vi "SE Initialization VI.vi"(8 "error in (no error)":errorcluster, 10 "Custom XML":string, 11 "Device Item Ref in":T1 format="%.0x") -> (0 "error out":errorcluster, 3 "Device Item Ref out":T1 format="%.0x")   [LabVIEW 2012, in "PXImc System Explorer.lvlib"]
uses:
  PXImc System Explorer.lvlib
  <vilib>/NI Veristand/Custom Device API/Custom Device Item Ref.ctl
  <vilib>/NI Veristand/Custom Device API/Custom Device Channel Type.ctl
  Shared/Channel.ctl
  Shared/Constants.vi
  <vilib>/dlg_ctls.llb/Space Constant.vi
  Shared/PXImc Shared.lvlib
  <vilib>/NI Veristand/Custom Device API/Custom Device API.lvlib
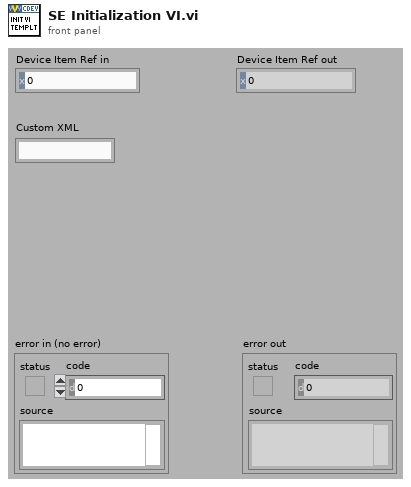
[diagram p1: front panel]
types:
  T1 = typedef "Custom Device API.lvlib/Custom Device Item Ref.ctl" = u64
  T2 = typedef "Custom Device API.lvlib/Custom Device Channel Type.ctl" = enum16{"Input", "Output"}
  T3 = typedef "PXImc Shared.lvlib/Channel.ctl" = cluster{"Name":string, "Units":string, "Default":dbl, "Description":string}
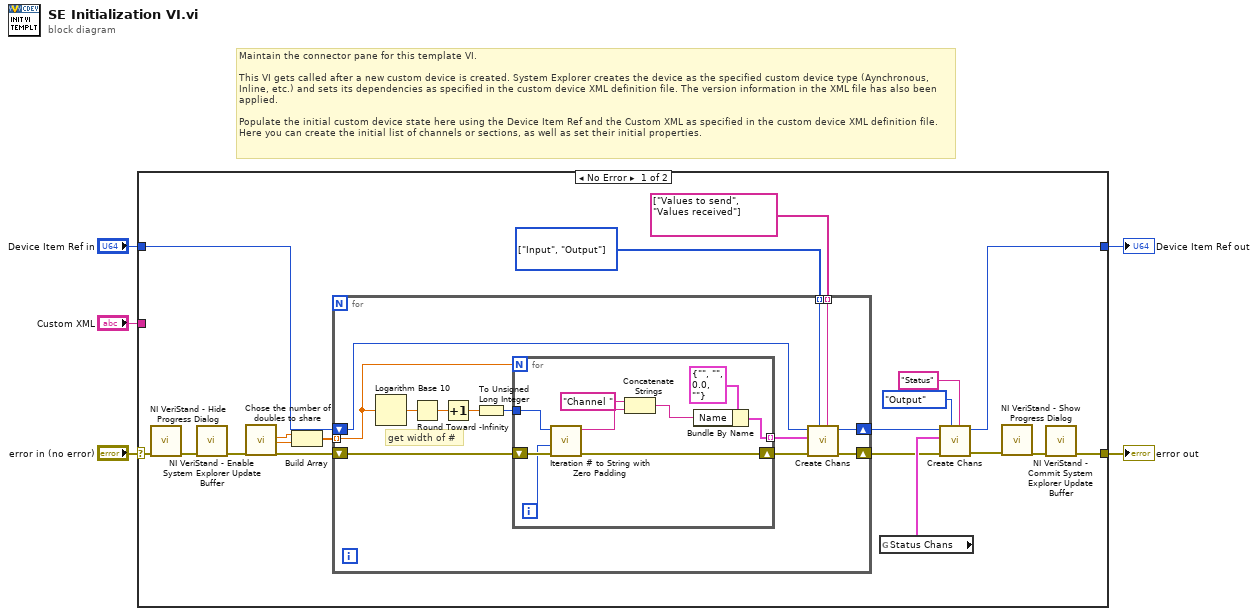
[diagram p0: block diagram]
diagram:
  # "Maintain the connector pane for this template VI.\n\nThis VI gets called after a new custom device is created. System Explorer creates the device as the specified custom device type (Aynchronous, Inline, etc.) and sets its dependencies as specified in the custom device XML definition file. The version information in the XML file has also been applied.\n\nPopulate the initial custom device state here using the Device Item Ref and the Custom XML as specified in the custom device XML definition file. Here you can create the initial list of channels or sections, as well as set their initial properties."
  n1 = case shown="No Error" "error in (no error)" {
    selector: "error in (no error)" -> [w17 w48]
    tunnel: [w12 w48] -> w5
    tunnel: [w24 w47] -> w3
    tunnel: "Device Item Ref in" -> [w10 w47]
    tunnel: "Custom XML" -> [_ _]
    frame No Error {
      w7 = T2[] [enum."Input", enum."Output"] items=["Input", "Output"]
      n2 = call <vilib>:"NI VeriStand - Hide Progress Dialog.vi"("error in (no error)"=w17) -> ("error out"=w16:errorcluster)  [unwired: 10 in]
      n3 = call <vilib>:"NI VeriStand - Enable System Explorer Update Buffer.vi"("error in (no error)"=w16) -> ("error out"=w15:errorcluster)  [unwired: 10 in]
      n4 = call "Chose the number of doubles to share"("error in (no error)"=w15) -> ("Doubles to receive"=w20:dbl, "Doubles to send"=w21:dbl, "error out"=w18:errorcluster)  [unwired: 15 in, 1 out]
      n5 = Build Array(w20, w21) -> (w19:dbl[])
      n6 = for {
        tunnel: w19 -> [w26] mode=indexing
        shift-right: [w36] -> w11
        shift-left: w18 -> [w37]
        shift-right: [w33] -> w9
        shift-left: w10 -> [w34]
        tunnel: string[] ["Values to send", "Values received"] -> [w31] mode=indexing
        tunnel: w7 -> [w30] mode=indexing
        # "get width of #"
        n7 = Logarithm Base 10(1:w26) -> (0:w27:dbl)
        n8 = Round Toward -Infinity(1:w27) -> (0:w28:dbl)
        n9 = Increment(x=w28) -> (x+1=w29:dbl)
        n10 = To Unsigned Long Integer(number=w29) -> (unsigned 32bit integer=w25:u32)
        n11 = for {
          N: w26 -> [_]
          shift-right: [w41] -> w35
          shift-left: w37 -> [w44]
          tunnel: [w45] -> w32 mode=indexing
          tunnel: w25 -> [w43]
          i -> [w42]
          n12 = call "Iteration # to String with Zero Padding.vi"("error in (no error)"=w44, "Current #"=w42, "Width"=w43) -> ("error out"=w41:errorcluster, "String"=w39:string)  [unwired: 7 in]
          n13 = Concatenate Strings("Channel " ("string"), w39) -> (w38:string)
          n14 = Bundle By Name(cluster=T3 {"Name"="", "Units"="", "Default"=0.0, "Description"=""} ("Channel"), "Name"=w38) -> (w45:T3)
        }
        n15 = call "Create Chans.vi"("New Section Name (none)"=w31, "Type"=w30, "error in (no error)"=w35, "Channels"=w32, "Section Ptr"=w34) -> ("error out"=w36:errorcluster, "Section Ptr dup"=w33:T1)  [unwired: 5 in]
      }
      n16 = global read "Constants.vi" "Status Chans"() -> (w23:T3[])
      n17 = call "Create Chans.vi"("New Section Name (none)"="Status", "Type"=Custom_Device_Channel_Type."Output", "error in (no error)"=w11, "Channels"=w23, "Section Ptr"=w9) -> ("error out"=w14:errorcluster, "Section Ptr dup"=w24:T1)  [unwired: 5 in]
      n18 = call <vilib>:"NI VeriStand - Show Progress Dialog.vi"("error in (no error)"=w14) -> ("error out"=w13:errorcluster)  [unwired: 10 in]
      n19 = call <vilib>:"NI VeriStand - Commit System Explorer Update Buffer.vi"("error in (no error)"=w13) -> ("error out"=w12:errorcluster)  [unwired: 10 in]
    }
    frame Error {
    }
  }
  "error out" <- w5
  "Device Item Ref out" <- w3
